vi "uc480_SubVI_Example_Is_XS.vi"(8 "Error In":errorcluster, 11 ".NET (Reference)":refnum<k24>) -> (0 "Error Out":errorcluster, 2 "BoardType":i32(ring)=1 items=["FALCON"=1, "EAGLE"=2, "FALCON2"=3, "FALCON_PLUS"=7, "FALCON_QUATTRO"=9, "FALCON_DUO"=10, "EAGLE_QUATTRO"=11, "EAGLE_DUO"=12, "Usb, Usb_SE, Usb_RE"=64, "Usb_ME"=65, "Usb_LE"=66, "Usb_XS"=67, "Usb_ML"=69, "Usb3_LE"=98, "Usb3_CP"=100, "Usb3_ML"=101, "Eth, Eth_HE"=128, "Eth_SE, Eth_RE"=129, "Eth_CP"=132, "Eth_SEP, Eth_REP"=134, "Eth_LEET"=135, "Eth_TE"=136], 3 "IsXS":bool)   [LabVIEW 2016]
uses:
  D:/Fabrizio/Labview Projects/IR OPO Controller/Branches/Schwarzschild version/uc480DotNet.dll
  uc480DotNet.dll
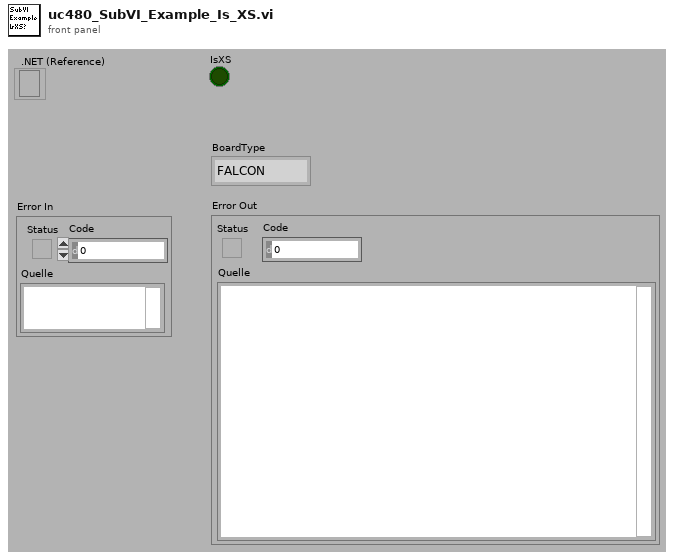
[diagram p1: front panel]
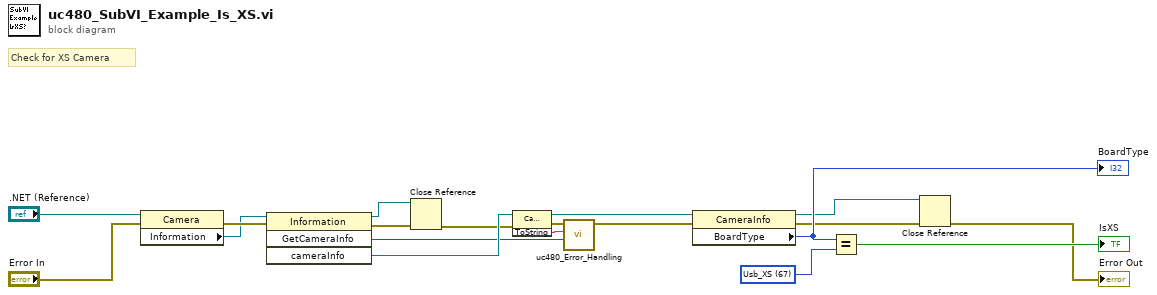
[diagram p0: block diagram]
diagram:
  w14 = 67 items=["FALCON"=1, "EAGLE"=2, "FALCON2"=3, "FALCON_PLUS"=7, "FALCON_QUATTRO"=9, "FALCON_DUO"=10, "EAGLE_QUATTRO"=11, "EAGLE_DUO"=12, "Usb, Usb_SE, Usb_RE"=64, "Usb_ME"=65, "Usb_LE"=66, "Usb_XS"=67, "Usb_ML"=69, "Usb3_LE"=98, "Usb3_CP"=100, "Usb3_ML"=101, "Eth, Eth_HE"=128, "Eth_SE, Eth_RE"=129, "Eth_CP"=132, "Eth_SEP, Eth_REP"=134, "Eth_LEET"=135, "Eth_TE"=136] ("BoardType")
  # "Check for XS Camera"
  n1 = property class="Camera"(reference=".NET (Reference)", error in="Error In") -> (error out=w17:errorcluster, "Information"=w16:refnum<k24>)  [unwired: 1 out]
  n2 = invoke class="Information" method="GetCameraInfo"(reference=w16, error in=w17) -> (reference out=w1:refnum<k24>, error out=w3:errorcluster, "GetCameraInfo"=w7:i32, "cameraInfo"=w10:refnum<k24>)  [unwired: 2 in]
  n3 = Close Reference(reference=w1, error in (no error)=w3) -> (error out=w2:errorcluster)
  n4 = invoke class="CameraInfo" method="ToString"(reference=w10, error in=w2) -> (reference out=w9:refnum<k24>, error out=w11:errorcluster, "ToString"=w12:string)  [unwired: 1 in]
  n5 = call "uc480_Error_Handling.vi"("Error Code"=w7, "Error String"=w12, "Error In"=w11) -> ("Error Out"=w8:errorcluster)  [unwired: 8 in]
  n6 = property class="CameraInfo"(reference=w9, error in=w8) -> (reference out=w4:refnum<k24>, error out=w6:errorcluster, "BoardType"=w15:i32)
  "BoardType" <- w15
  n7 = Equal?(x=w15, y=w14) -> (x = y?=→"IsXS":bool)
  n8 = Close Reference(reference=w4, error in (no error)=w6) -> (error out=→"Error Out":errorcluster)
